vi "DlgConfirmCalcSummary.vi"(7 "Suffix":string, 8 "error in (no error)":errorcluster, 10 "Path":path, 11 "PMUConfig":T1) -> (0 "error out":errorcluster, 1 "Summary Data Excel File":path, 2 "Path":path, 3 "PMUConfig":T1)   [LabVIEW 2014]
uses:
  typedef/PMUConfig.ctl
  typedef/appState.ctl
panel:
  in  "BtnAbort":bool
  in  "BtnSkip":bool
  in  "BtnChange":bool
  in  "BtnProcess":bool
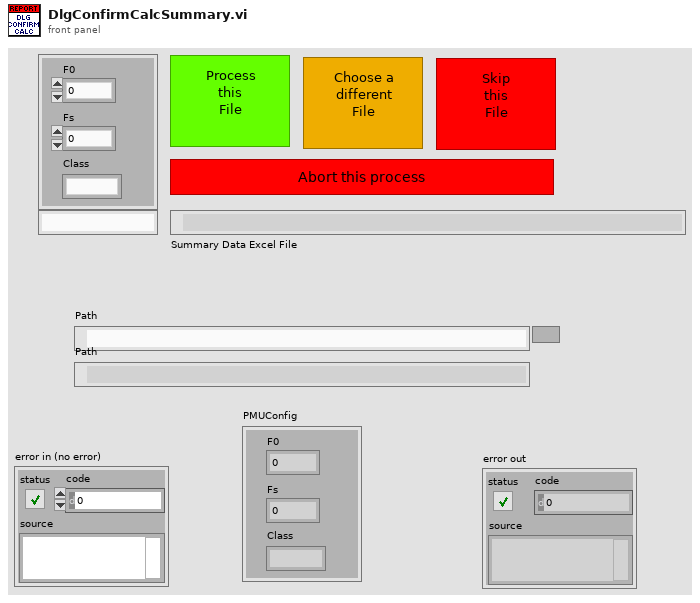
[diagram p1: front panel]
types:
  T1 = typedef "PMUConfig.ctl" = cluster{"Class":string, "Fs":dbl, "F0":dbl}
  T2 = typedef "appState.ctl" = enum16{"init", "processUI", "exit"}
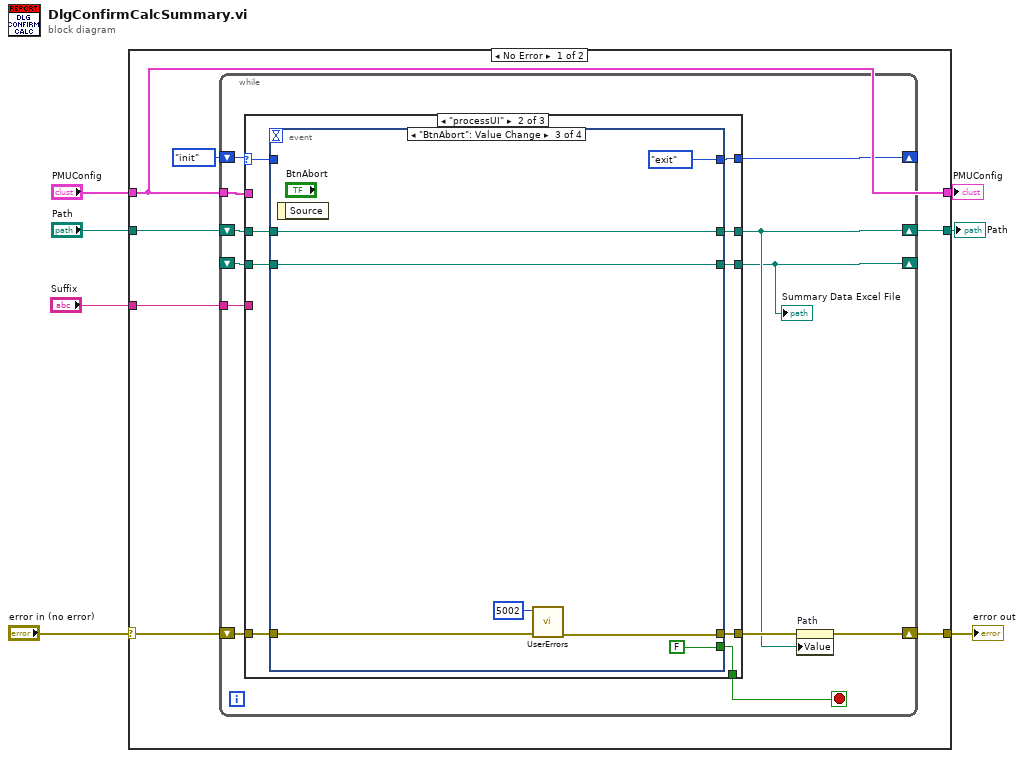
[diagram p0: block diagram]
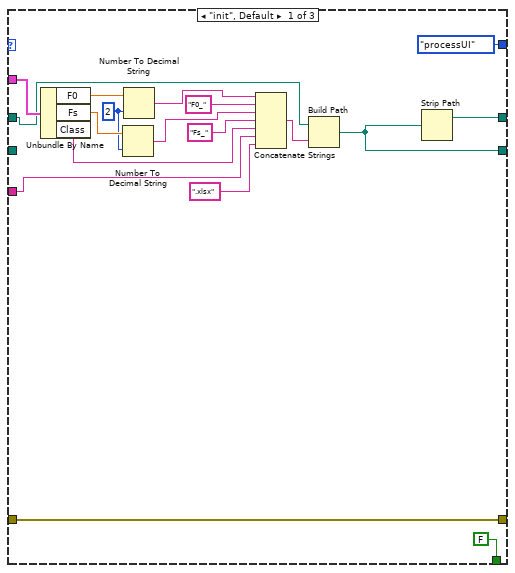
[diagram p2: hidden frame]
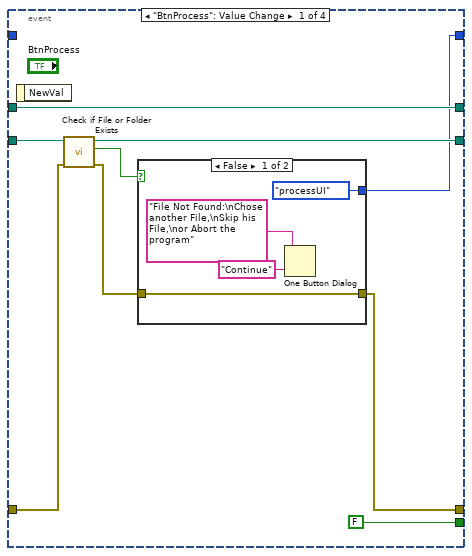
[diagram p3: hidden frame]
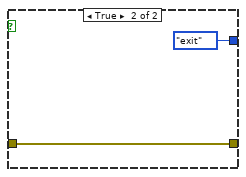
[diagram p4: hidden frame]
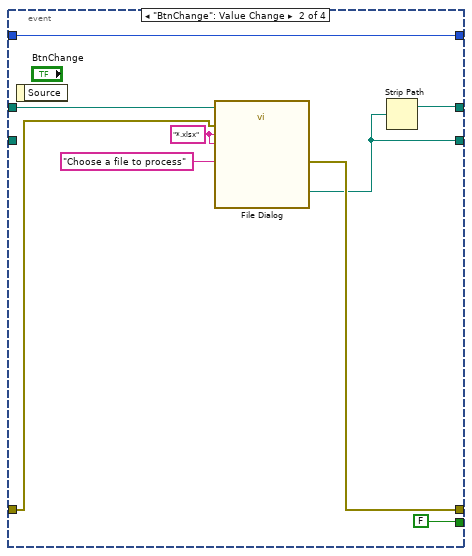
[diagram p5: hidden frame]
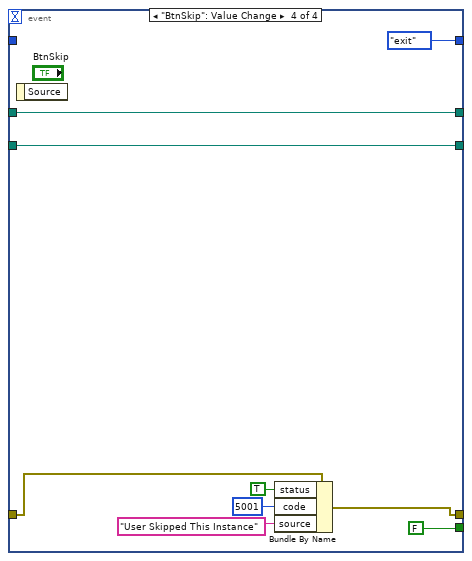
[diagram p6: hidden frame]
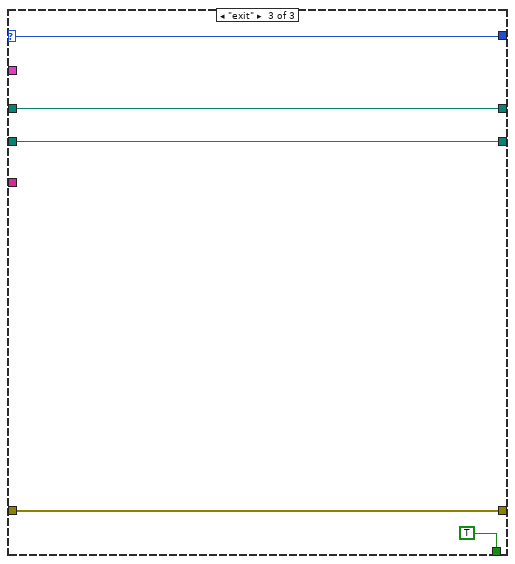
[diagram p7: hidden frame]
diagram:
  n1 = case shown="No Error" "error in (no error)" {
    selector: "error in (no error)" -> [w12 w101]
    tunnel: [w11 w101] -> w6
    tunnel: "PMUConfig" -> [w9 w99]
    tunnel: "Path" -> [w13 w100]
    tunnel: [w10 w100] -> w3
    tunnel: [w9 w99] -> w2
    tunnel: "Suffix" -> [w8 _]
    frame No Error {
      n2 = while {
        tunnel: w9 -> [w25]
        shift-right: [w18] -> w11
        shift-left: w12 -> [w23]
        shift-right: [w20] -> _
        shift-left: appState."init" ("AppState") -> [w26]
        shift-right: [w17] -> w10
        shift-left: w13 -> [w24]
        shift-right: [w16] -> _
        shift-left: _ -> [w21]
        tunnel: w8 -> [w15]
        stop <- w22 stop-if-true
        n3 = case shown="\"processUI\"" w26 {
          selector: w26 -> [_ w52 w98]
          tunnel: w25 -> [w43 _ _]
          tunnel: w24 -> [w33 w50 w96]
          tunnel: w23 -> [w44 w46 w94]
          tunnel: [w44 w45 w94] -> w19
          tunnel: [w30 w47 w95] -> w16
          tunnel: [FALSE w53 TRUE] -> w22
          tunnel: [w29 w49 w96] -> w17
          tunnel: w21 -> [_ w48 w95]
          tunnel: [appState."processUI" ("AppState") w51 w98] -> w20
          tunnel: w15 -> [w28 _ _]
          frame "init", Default {
            w39 = i16 2 ("width (-)")
            n4 = Unbundle By Name(w43) -> ("F0"=w41:dbl, "Fs"=w40:dbl, "Class"=w34:string)
            n5 = Number To Decimal String(number=w40, width (-)=w39) -> (decimal integer string=w35:string)
            n6 = Number To Decimal String(number=w41, width (-)=w39) -> (decimal integer string=w36:string)
            n7 = Concatenate Strings(w36, "F0_" ("string"), w35, "Fs_" ("string"), w34, w28, ".xlsx" ("string")) -> (w32:string)
            n8 = Build Path(base path=w33, name or relative path=w32) -> (appended path=w30:path)
            n9 = Strip Path(path=w30) -> (stripped path=w29:path)  [unwired: 1 out]
          }
          frame "processUI" {
            n10 = event shown="[2] \"BtnAbort\": Value Change" {
              selector: _ -> [_ _ _ _]
              dyn-events: _ -> [_ _ _ _]
              timeout: _ -> [_ _ _ _]
              tunnel: [FALSE FALSE FALSE FALSE] -> w53
              tunnel: w52 -> [_ w77 _ _]
              tunnel: [w54 w77 appState."exit" ("AppState") appState."exit" ("AppState")] -> w51
              tunnel: w50 -> [w61 w76 w80 w92]
              tunnel: [w61 w69 w80 w92] -> w49
              tunnel: [w59 w70 w79 w91] -> w47
              tunnel: w48 -> [w60 _ w79 w91]
              tunnel: w46 -> [w56 w73 w82 w85]
              tunnel: [w55 w72 w81 w86] -> w45
              event "BtnProcess": Value Change {
                n11 = event-data() -> ()  [unwired: 1 in, 1 out]
                n12 = call <vilib>:"Check if File or Folder Exists.vi"("error in (no error)"=w56, "path"=w60) -> ("error out"=w57:errorcluster, "file or folder exists?"=w58:bool, "dup path"=w59:path)  [unwired: 7 in]
                n13 = case shown="False" w58 {
                  tunnel: w57 -> [w64 w68]
                  tunnel: [w64 w68] -> w55
                  tunnel: [appState."processUI" ("AppState") appState."exit" ("AppState")] -> w54
                  frame False {
                    n14 = One Button Dialog(message="File Not Found:\nChose another File,\nSkip his File,\nor Abort the program", button name ("OK")="Continue") -> ()  [unwired: 1 out]
                  }
                  frame True {
                  }
                }
              }
              event "BtnChange": Value Change {
                w75 = "*.xlsx" ("pattern (all files)")
                n15 = event-data() -> ()  [unwired: 1 in, 1 out]
                n16 = call "File Dialog"("start path"=w76, "prompt"="Choose a file to process", "error in"=w73, "pattern (all files)"=w75, "pattern label"=w75) -> ("selected path"=w70:path, "error out"=w72:errorcluster)  [unwired: 7 in, 2 out]
                n17 = Strip Path(path=w70) -> (stripped path=w69:path)  [unwired: 1 out]
              }
              event "BtnAbort": Value Change {
                n18 = event-data() -> ()  [unwired: 1 in, 1 out]
                n19 = call "UserErrors.vi"("error in (no error)"=w82, "[error code] (0)"=5002) -> ("error out"=w81:errorcluster)  [unwired: 9 in]
              }
              event "BtnSkip": Value Change {
                n20 = event-data() -> ()  [unwired: 1 in, 1 out]
                n21 = Bundle By Name(cluster=w85, "status"=TRUE, "code"=5001 ("[error code] (0)"), "source"="User Skipped This Instance") -> (w86:errorcluster)
              }
            }
          }
          frame "exit" {
          }
        }
        "Summary Data Excel File" <- w16
        n22 = property on="Path" class="Path"(error in=w19, "Value"=w17) -> (error out=w18:errorcluster)  [unwired: 1 in, 1 out]
      }
    }
    frame Error {
    }
  }
  "PMUConfig" <- w2
  "error out" <- w6
  "Path" <- w3
